vi "Set VI Icon Colour.vi"(6 "VI Path":path, 7 "Colour string":string, 8 "error in (no error)":errorcluster, 10 "ImageData (Test IP only)":T1) -> (0 "error out":errorcluster, 2 "ImageData (Test OP only)":T1)   [LabVIEW 2018]
doc: "Changes the background colour of the vi icon to match the colour requested (plan is to make this match the data type of the assert vi)"
uses:
  <vilib>/picture/picture.llb/imagedata.ctl
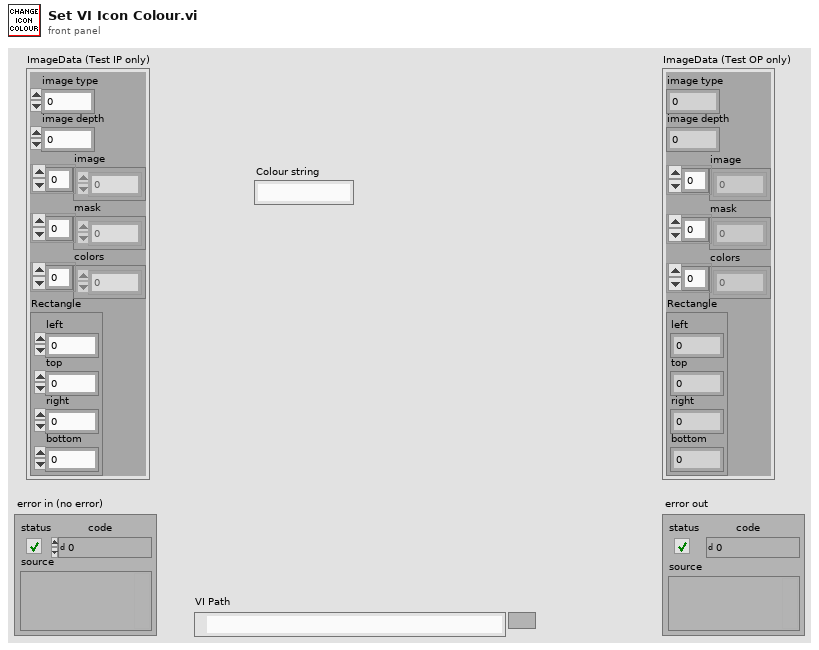
[diagram p1: front panel]
types:
  T1 = typedef "imagedata.ctl" = cluster{"image type":i32, "image depth":i32, "image":u8[], "mask":u8[], "colors":u32[], "Rectangle":cluster{"left":i16, "top":i16, "right":i16, "bottom":i16}}
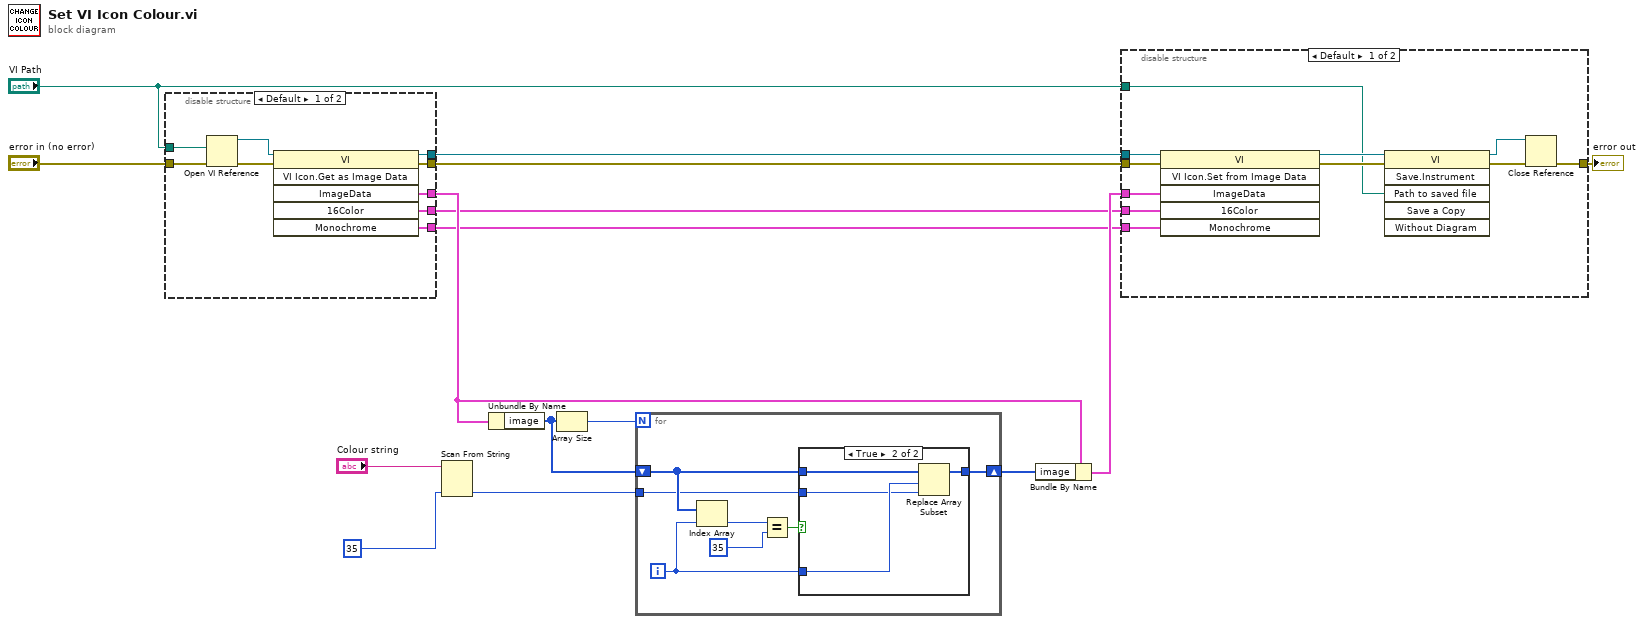
[diagram p0: block diagram]
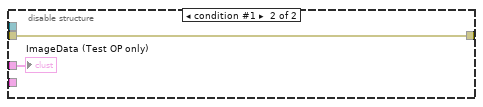
[diagram p3: hidden frame]
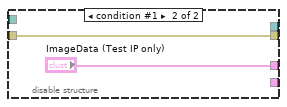
[diagram p4: hidden frame]
diagram:
  n1 = disable-structure shown="Default" {
    disable-tunnel: [w23 _] -> w15
    disable-tunnel: [w22 w26] -> w14
    disable-tunnel: "error in (no error)" -> [w20 w26]
    disable-tunnel: [w19 "ImageData (Test IP only)"] -> w12
    disable-tunnel: [w18 _] -> w10
    disable-tunnel: [w17 _] -> w9
    disable-tunnel: "VI Path" -> [w16 _]
    frame condition #0 (active) {
      n2 = Open VI Reference(vi path=w16, error in (no error)=w20) -> (vi reference=w24:refnum<vi>, error out=w21:errorcluster)  [unwired: 4 in]
      n3 = invoke class="VI" method="VI Icon.Get as Image Data"(reference=w24, error in=w21) -> (reference out=w23:refnum<vi>, error out=w22:errorcluster, "ImageData"=w19:T1, "16Color"=w18:T1, "Monochrome"=w17:T1)  [unwired: 4 in, 1 out]
    }
    frame condition #1 {
    }
  }
  n4 = Scan From String(input string="Colour string", default 1=u8 35 ("y")) -> (output 1=w2:u8)  [unwired: 3 in, 3 out]
  n5 = Unbundle By Name(w12) -> ("image"=w5:u8[])
  n6 = Array Size(array=w5) -> (size(s)=w4:i32)
  n7 = for {
    N: w4 -> [_]
    shift-right: [w29] -> w6
    shift-left: w5 -> [w31]
    tunnel: w2 -> [w27]
    i -> [w30]
    n8 = Index Array(array=w31, index=w30) -> (element=w32:u8)
    n9 = Equal?(x=w32, y=u8 35) -> (x = y?=w28:bool)
    n10 = case shown="True" w28 {
      tunnel: w31 -> [w34 w38]
      tunnel: w30 -> [_ w36]
      tunnel: [w34 w37] -> w29
      tunnel: w27 -> [_ w35]
      frame False {
      }
      frame True {
        n11 = Replace Array Subset(array=w38, new element=w35, index=w36) -> (w37:u8[])
      }
    }
  }
  n12 = Bundle By Name(cluster=w12, "image"=w6) -> (w11:T1)
  n13 = disable-structure shown="Default" {
    disable-tunnel: w15 -> [w49 _]
    disable-tunnel: w14 -> [w48 w51]
    disable-tunnel: w11 -> [w47 w50]
    disable-tunnel: w10 -> [w46 _]
    disable-tunnel: w9 -> [w45 _]
    disable-tunnel: "VI Path" -> [w42 _]
    disable-tunnel: [w39 w51] -> w7
    frame condition #0 (active) {
      n14 = invoke class="VI" method="VI Icon.Set from Image Data"(reference=w49, error in=w48, "ImageData"=w47, "16Color"=w46, "Monochrome"=w45) -> (reference out=w44:refnum<vi>, error out=w43:errorcluster)  [unwired: 1 in, 4 out]
      n15 = invoke class="VI" method="Save.Instrument"(reference=w44, error in=w43, "Path to saved file"=w42) -> (reference out=w41:refnum<vi>, error out=w40:errorcluster)  [unwired: 3 in, 4 out]
      n16 = Close Reference(reference=w41, error in (no error)=w40) -> (error out=w39:errorcluster)
    }
    frame condition #1 {
      "ImageData (Test OP only)" <- w50
    }
  }
  "error out" <- w7
